vi "Write ADS State.vi"(8 "error in (no error)":errorcluster, 10 "ADS State":i16(ring) items=["Invalid", "Idle", "Reset", "Init", "Start", "Run", "Stop", "SaveConfig", "LoadConfig", "PowerFailure", "PowerGood", "Error", "Shutdown", "Suspend", "Resume", "Config", "Reconfig", "Stopping, Maxstates", "Incompatible", "Exception"], 11 "TwinCAT ADS in":refnum<class "TwinCAT ADS.lvclass">) -> (0 "error out":errorcluster, 3 "TwinCAT ADS out":refnum<class "TwinCAT ADS.lvclass">)   [LabVIEW 2018, in "TwinCAT ADS.lvclass"]
uses:
  TwinCAT ADS.lvclass
  TwinCAT ADS.lvclass/TwinCAT ADS.ctl
  TwinCAT.Ads
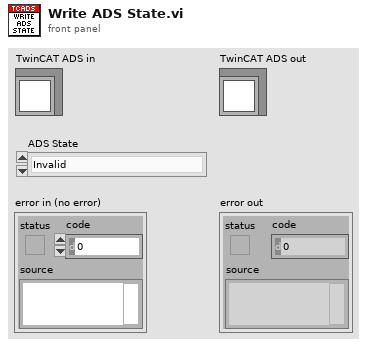
[diagram p1: front panel]
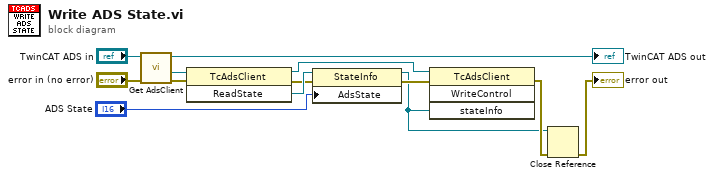
[diagram p0: block diagram]
diagram:
  n1 = call "Get AdsClient.vi"("error in (no error)"="error in (no error)", "TwinCAT ADS in"="TwinCAT ADS in") -> ("error out"=w7:errorcluster, ".NET TcAdsClient"=w6:refnum<k24>, "TwinCAT ADS out"=→"TwinCAT ADS out":refnum<class "TwinCAT ADS.lvclass">)  [unwired: 7 in]
  n2 = invoke class="TcAdsClient" method="ReadState"(reference=w6, error in=w7) -> (reference out=w5:refnum<k24>, error out=w8:errorcluster, "ReadState"=w9:refnum<k24>)  [unwired: 1 in]
  n3 = property class="StateInfo"(reference=w9, error in=w8, "AdsState"="ADS State") -> (reference out=w1:refnum<k24>, error out=w10:errorcluster)
  n4 = invoke class="TcAdsClient" method="WriteControl"(reference=w5, error in=w10, "stateInfo"=w1) -> (error out=w3:errorcluster)  [unwired: 1 in, 3 out]
  n5 = Close Reference(reference=w1, error in (no error)=w3) -> (error out=→"error out":errorcluster)
